vi "LM model function and gradient (2-Exp + IRF) v2.vi"(3 "output control":T1, 4 "data":variant, 5 "X":dbl[](array[numeric]), 6 "a":dbl[](array[numeric])) -> (0 "error out":errorcluster, 1 "f'(X,a)":dbl[][](array[numeric]), 2 "f(X,a)":dbl[](array[numeric]))   [LabVIEW 2021, in "Fits.lvlib"]
doc: "This template is the starting point for creating a model function to be passed to the Nonlinear Curve Fit.vi."
uses:
  Fits.lvlib
  <vilib>/gmath/NumericalOptimization/LM_output select.ctl
  011e43be-0096-45db-939d-702c55b52cee.vi
  <vilib>/Analysis/2dsp.llb/1D Convolution (DBL).vi
  d8a27459-d410-48d4-9d81-9035e4d4d056.vi
  <vilib>/Analysis/NI_AALPro.lvlib
  Error/Error.lvlib
  <vilib>/gmath/NI_Gmath.lvlib
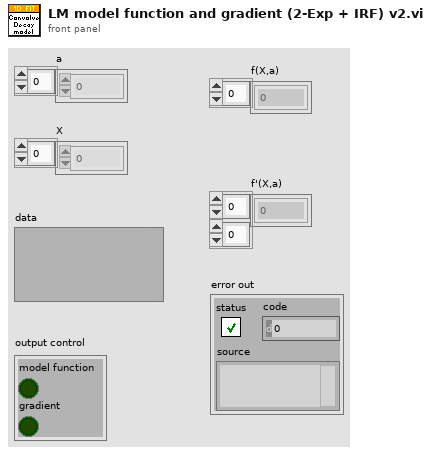
[diagram p1: front panel]
types:
  T1 = typedef "NI_Gmath.lvlib/LM_output select.ctl" = cluster{"model function":bool, "gradient":bool}
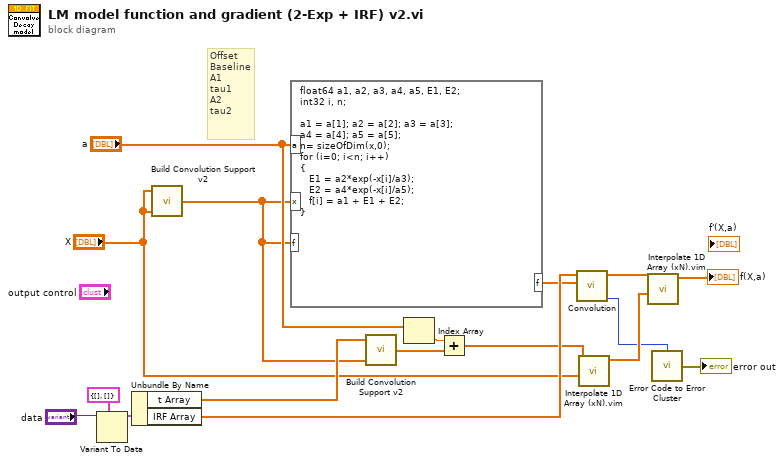
[diagram p0: block diagram]
diagram:
  # "Offset\nBaseline\nA1\ntau1\nA2\ntau2"
  n1 = Variant To Data(type=cluster{"t Array":dbl[], "IRF Array":dbl[]} {"t Array"=[], "IRF Array"=[]} ("IRF"), Variant="data") -> (data=w15:cluster{"t Array":dbl[], "IRF Array":dbl[]})  [unwired: 1 in, 1 out]
  n2 = Unbundle By Name(w15) -> ("t Array"=w9:dbl[], "IRF Array"=w14:dbl[])
  n3 = call "Build Convolution Support v2.vi"("X Array 2"="X", "X Array 1"="X") -> ("X Arrays Convolution Support"=w3:dbl[])  [unwired: 3 in]
  n4 = formula code="float64 a1, a2, a3, a4, a5, E1, E2;\nint32 i, n;\n\na1 = a[1]; a2 = a[2]; a3 = a[3];\na4 = a[4]; a5 = a[5];\nn= sizeOfDim(x,0);\nfor (i=0; i<n; i++)\n{\n   E1 = a2*exp(-x[i]/a3);\n   E2 = a4*exp(-x[i]/a5);\n   f[i] = a1 + E1 + E2;\n}"("a"="a", "x"=w3, "f"=w3) -> ("f"=w13:dbl[])
  n5 = call "Build Convolution Support v2.vi"("X Array 2"=w3, "X Array 1"=w9) -> ("X Arrays Convolution Support"=w7:dbl[])  [unwired: 3 in]
  n6 = Index Array(array="a") -> (element=w5:dbl)  [unwired: 1 in]
  n7 = Add(x=w5, y=w7) -> (x+y=w6:dbl[])
  n8 = call-poly <vilib>:"Convolution.vi"("Y"=w13, "X"=w14) -> ("error"=w2:i32, "X * Y"=w12:dbl[])  [unwired: 8 in]
  n9 = call "Interpolate 1D Array (xN).vim"("Interpolated Indices"="X", "Y"=w6) -> ("Interpolated Y"=w11:dbl[])  [unwired: 9 in]
  n10 = call "Interpolate 1D Array (xN).vim"("Interpolated Indices"=w11, "Y"=w12) -> ("Interpolated Y"=→"f(X,a)":dbl[])  [unwired: 9 in]
  n11 = call "Error Code to Error Cluster.vi"("Error Code"=w2) -> ("Error Out"=→"error out":errorcluster)  [unwired: 14 in]
